vi "cic5_test.vi"() -> ()   [LabVIEW 2013]
uses:
  <vilib>/rvi/FXPMathLib/FxpConvert/subVIs/nifxpmath_Convert_SimConfig.ctl
  <vilib>/fxp/LVFixedPointQuantizationPolicyTypeDef.ctl
  <vilib>/fxp/LVFixedPointOverflowPolicyTypeDef.ctl
  <vilib>/rvi/FXPMathLib/FxpConvert/simVIs/DllFxpConvertTemp_sub.vi
  <vilib>/rvi/FXPMathLib/FxpInterpret/XNode/nifxpmath_Interpret.xnode
  <vilib>/rvi/FXPMathLib/FxpConvert/XNode/nifxpmath_Convert.xnode
panel:
  out "Array 4":fxp<+/-,20,16>[](array[numeric])
  out "Array 3":bool[](array[boolean])
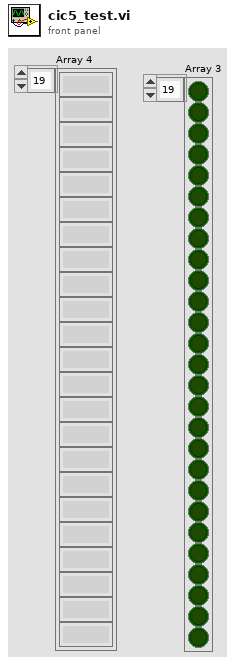
[diagram p1: front panel]
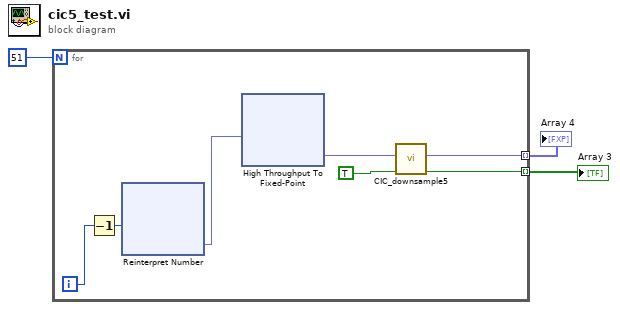
[diagram p0: block diagram]
diagram:
  n1 = for {
    N: 51 -> [_]
    tunnel: [w8] -> w2 mode=indexing
    tunnel: [w7] -> w1 mode=indexing
    i -> [w10]
    n2 = Decrement(x=w10) -> (x-1=w4:i32)
    n3 = xnode "Reinterpret Number"("x"=w4) -> ("y"=w6:fxp<+/-,32,32>)
    n4 = xnode "High Throughput To Fixed-Point"("x"=w6) -> ("y"=w5:fxp<+/-,20,16>)
    n5 = call "CIC_downsample5.vi"("valid in"=TRUE, "din"=w5) -> ("valid out"=w7:bool, "dout"=w8:fxp<+/-,20,16>)  [unwired: 8 in]
  }
  "Array 3" <- w1
  "Array 4" <- w2
